vi "voltage.vi"(2 "divider":dbl, 3 "voltage \nreferences":enum16{"2,56", "5,00"}(ring), 4 "id pin":T1(ring), 5 "connection in":refnum<k31>) -> (0 "voltage":dbl, 1 "connection out":refnum<k31>)   [LabVIEW 2012]
panel:
  out "command id":u8
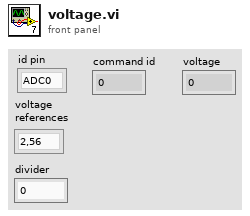
[diagram p1: front panel]
types:
  T1 = enum16{"ADC0", "ADC1", "ADC2", "ADC3", "ADC4", "ADC5", "ADC6", "ADC7"}
  T2 = cluster{"param":u64, "count":i32, "name":string}[]
  T3 = cluster{"received values[0]":u8, "received values[1]":u8, "received values[2]":u8, "received values[3]":u8, "received values[4]":u8, "received values[5]":u8, "received values[6]":u8, "received values[7]":u8, "received values[8]":u8}
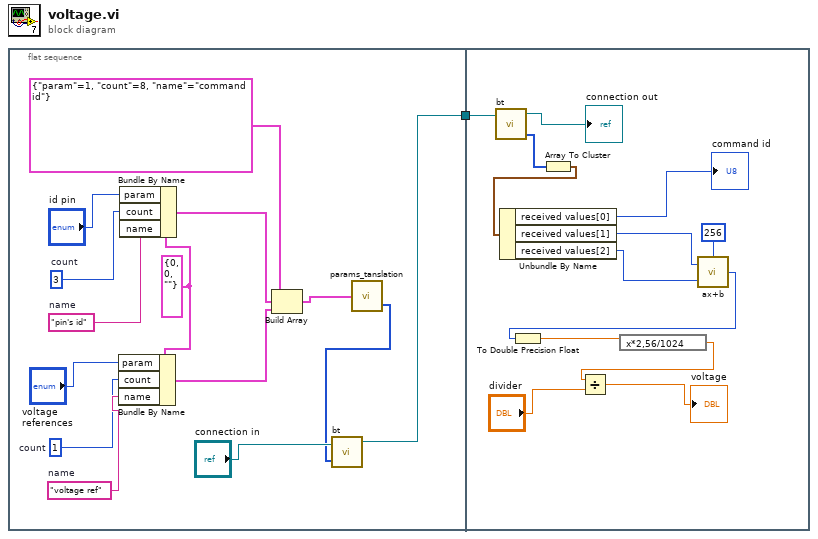
[diagram p0: block diagram]
diagram:
  n1 = flat-sequence {
    tunnel: [w10] -> w1
    tunnel: w1 -> [w28]
    frame #0 {
      w8 = 1  # count
      w9 = "voltage ref"  # name
      w13 = u8 3  # count
      w14 = "pin's id"  # name
      w7 = cluster{"param":u64, "count":u8, "name":string} {"param"=0, "count"=0, "name"=""} ("Cluster")
      n2 = Bundle By Name(cluster=w7, "param"="voltage \nreferences", "count"=w8, "name"=w9) -> (w3:cluster{"param":u64, "count":u8, "name":string})
      n3 = Bundle By Name(cluster=w7, "param"="id pin", "count"=w13, "name"=w14) -> (w4:cluster{"param":u64, "count":u8, "name":string})
      n4 = Build Array(cluster{"param":i32, "count":i32, "name":string} {"param"=1, "count"=8, "name"="command id"} ("Cluster"), w4, w3) -> (w2:T2)
      n5 = call "params_tanslation.vi"("params"=w2) -> ("tablica charow (u8)"=w11:u8[])  [unwired: 1 out]
      n6 = call "bt.vi"("connection in"="connection in", "sending command"=w11) -> ("connection out"=w10:refnum<k31>)  [unwired: 2 out]
    }
    frame #1 {
      n7 = call "bt.vi"("connection in"=w28) -> ("connection out"=→"connection out":refnum<k31>, "received values"=w19:u8[])  [unwired: 1 in, 1 out]
      n8 = Array To Cluster(array=w19) -> (cluster=w20:T3)
      n9 = Unbundle By Name(w20) -> ("received values[0]"=→"command id":u8, "received values[1]"=w22:u8, "received values[2]"=w23:u8)
      n10 = call "ax+b.vi"("x"=256, "b"=w23, "a"=w22) -> ("y"=w25:i32)
      n11 = To Double Precision Float(number=w25) -> (double precision float=w26:dbl)
      n12 = expression code="x*2,56/1024"(w26) -> (w18:dbl)
      n13 = Divide(x=w18, y="divider") -> (x/y=→"voltage":dbl)
    }
  }
